vi "gentec-M-Link.Example.vi"() -> ()   [LabVIEW 2014, in "gentec-M-Link - Driver.lvlib"]
uses:
  gentec-M-Link - Driver.lvlib
  Driver/Type Defs/gentec-M-Link.Waveform Averages.ctl
  Driver/Type Defs/gentec-M-Link.Range Queries.ctl
  Driver/Type Defs/gentec-M-Link.Range.ctl
  Driver/Type Defs/gentec-M-Link.Head Attributes.ctl
  Driver/Type Defs/gentec-M-Link.Sensor Type.ctl
  Driver/Type Defs/gentec-M-Link.Trigger Polarity.ctl
  Driver/Type Defs/gentec-M-Link.Trigger Source.ctl
  Driver/Type Defs/gentec-M-Link.Queries with String Answers.ctl
  Driver/Type Defs/gentec-M-Link.Measurement Mode.ctl
panel:
  in  "VISA resource":refnum<visa-resource-name>="visa://pppc069/COM6"
  in  "Action":u32(colorbox)
  in  "Tab Control":T1(tab)
  in  "Get Head connected":bool caption="Check: Head connected?"
  in  "String to send":string
  out "Timeout Test":bool caption="Timeout"
  out "Data read Test":string caption="Data read"
  out "Timeout Head connected":bool caption="Timeout"
  out "Data read Head connected":string caption="Data read"
  out "Head connected?":bool
  in  "Set Block Signal":bool
  in  "Query Head Attributes":bool
  out "Head Attributes":T2={"Firmware"="1.00.00\r\n", "Head Type"="PE3B-Si\r\n", "Head S/N"=501232, "min. Wavelength"=200.0, "max. Wavelength"=1060.0, "Wavelength"=200.0, "Area"=0.0, "Range"=0, "max. Range"=0} {"max. Range" items=["1f", "3f", "10f", "30f", "100f", "300f", "1p", "3p", "10p", "30p", "100p", "300p", "1n", "3n", "10n", "30n", "100n", "300n", "1u", "3u", "10u", "30u", "100u", "300u", "1m", "3m", "10m", "30m", "100m", "300m", "1", "3", "10", "30", "100", "300", "1K", "3K", "10K", "30K", "100K", "300K", "1M", "3M", "10M", "30M", "100M", "300M"]; "Range" items=["1f", "3f", "10f", "30f", "100f", "300f", "1p", "3p", "10p", "30p", "100p", "300p", "1n", "3n", "10n", "30n", "100n", "300n", "1u", "3u", "10u", "30u", "100u", "300u", "1m", "3m", "10m", "30m", "100m", "300m", "1", "3", "10", "30", "100", "300", "1K", "3K", "10K", "30K", "100K", "300K", "1M", "3M", "10M", "30M", "100M", "300M"]}
  out "Any Timeout head Attributes?":bool caption="Timeout"
  out "all Data read":string caption="Data read"
  out "Aswer":string caption="Answer"
  in  "Queries with String Answers":T4="VER"
  in  "Query Cal Lambda":bool
  out "Timeout Cal Lambda":bool caption="Timeout"
  out "Data read Cal Lambda":string caption="Data read"
  in  "Query Sensor Type":bool
  out "Timeout Sensor Type":bool caption="Timeout"
  out "Data read Sensor Type":string caption="Data read"
  out "Sensor Type":T5=2 items=["unknown", "Radiometer", "Joule Meter", "Optical Power", "Thermopyle Power"]
  out "Cal Lambda":i32
  out "Timeout Queries with String Answers":bool caption="Timeout"
  out "Data read  Queries with String Answers":string caption="Data read"
  in  "Get Waveform Averages":bool
  out "Timeout Get Waveform Averages":bool caption="Timeout"
  out "Data read Get Waveform Averages":string caption="Data read"
  in  "Set Waveform Averages":T6 items=["None", "2", "4", "8", "16", "32", "64", "128"]
  out "Timeout Set Waveform Averages":bool caption="Timeout"
  out "Data read Set Waveform Averages":string caption="Data read"
  out "ok Set Waveform Averages":bool caption="ok"
  out "Waveform Averages":T6 items=["None", "2", "4", "8", "16", "32", "64", "128"]
  in  "Set Zero":bool
  out "Range Set Zero":T3 caption="Range" items=["1f", "3f", "10f", "30f", "100f", "300f", "1p", "3p", "10p", "30p", "100p", "300p", "1n", "3n", "10n", "30n", "100n", "300n", "1u", "3u", "10u", "30u", "100u", "300u", "1m", "3m", "10m", "30m", "100m", "300m", "1", "3", "10", "30", "100", "300", "1K", "3K", "10K", "30K", "100K", "300K", "1M", "3M", "10M", "30M", "100M", "300M"]
  out "ok Set Zero":bool caption="ok"
  out "Data Read Set Zero":string caption="Data Read"
  out "Read Timeout Set Zero":bool caption="Timeout"
  out "Max Range Wavelength 2":dbl caption="Offset [V]"
  out "Current Range Wavelength 2":u32 caption="ADC Counts"
  out "Energy evolution":dbl(graph)
  in  "Get current measurement":bool
  out "Energy [J]":dbl format="%_3p"
  in  "Start or stop Data Flow":bool
  out "last measured Energy [J]":dbl format="%_3p"
  out "Success Stop Continuous Mode":bool caption="Success"
  out "Timeout Stop Continuous Mode":bool caption="Timeout"
  out "Data Read Continuous Mode":string caption="Data Read"
  out "Data Read Current Measurement":string
  out "Read Timeout Current Measurement":bool caption="Timeout"
  in  "Set Wavelength":u16 caption="Set Wavelength (nm)"
  out "Min Range Wavelength":T3 caption="Min Range" items=["1f", "3f", "10f", "30f", "100f", "300f", "1p", "3p", "10p", "30p", "100p", "300p", "1n", "3n", "10n", "30n", "100n", "300n", "1u", "3u", "10u", "30u", "100u", "300u", "1m", "3m", "10m", "30m", "100m", "300m", "1", "3", "10", "30", "100", "300", "1K", "3K", "10K", "30K", "100K", "300K", "1M", "3M", "10M", "30M", "100M", "300M"]
  out "Max Range Wavelength":T3 caption="Max Range" items=["1f", "3f", "10f", "30f", "100f", "300f", "1p", "3p", "10p", "30p", "100p", "300p", "1n", "3n", "10n", "30n", "100n", "300n", "1u", "3u", "10u", "30u", "100u", "300u", "1m", "3m", "10m", "30m", "100m", "300m", "1", "3", "10", "30", "100", "300", "1K", "3K", "10K", "30K", "100K", "300K", "1M", "3M", "10M", "30M", "100M", "300M"]
  out "Current Range Wavelength":T3 caption="Current Range" items=["1f", "3f", "10f", "30f", "100f", "300f", "1p", "3p", "10p", "30p", "100p", "300p", "1n", "3n", "10n", "30n", "100n", "300n", "1u", "3u", "10u", "30u", "100u", "300u", "1m", "3m", "10m", "30m", "100m", "300m", "1", "3", "10", "30", "100", "300", "1K", "3K", "10K", "30K", "100K", "300K", "1M", "3M", "10M", "30M", "100M", "300M"]
  out "Corrections Wavelength":bool caption="Corrections"
  out "Read Timeout Set Wavelength":bool caption="Timeout"
  out "Data Read Set Wavelength":string caption="Data Read"
  out "Error Set Wavelength":bool caption="Error"
  out "Min Lambda":i32
  out "Max Lambda":i32
  out "Data Read Set Head Attenuator":string caption="Data Read"
  out "Read Timeout Set Head Attenuator":bool caption="Timeout"
  in  "Set Head Attenuator":bool
  out "Data Read Set Range":string caption="Data Read"
  out "ok Set Autorange?":bool caption="ok?"
  out "Data Read Set Auto Range":string caption="Data Read"
  out "Read Timeout Set Auto Range":bool caption="Timeout"
  in  "Set Auto Range":bool
  in  "Get Range":T7="RNG"
  in  "Set Range":T3 items=["1f", "3f", "10f", "30f", "100f", "300f", "1p", "3p", "10p", "30p", "100p", "300p", "1n", "3n", "10n", "30n", "100n", "300n", "1u", "3u", "10u", "30u", "100u", "300u", "1m", "3m", "10m", "30m", "100m", "300m", "1", "3", "10", "30", "100", "300", "1K", "3K", "10K", "30K", "100K", "300K", "1M", "3M", "10M", "30M", "100M", "300M"]
  out "ok Set Range?":bool caption="ok?"
  out "Read Timeout Set Range":bool caption="Timeout"
  out "Range":T3 items=["1f", "3f", "10f", "30f", "100f", "300f", "1p", "3p", "10p", "30p", "100p", "300p", "1n", "3n", "10n", "30n", "100n", "300n", "1u", "3u", "10u", "30u", "100u", "300u", "1m", "3m", "10m", "30m", "100m", "300m", "1", "3", "10", "30", "100", "300", "1K", "3K", "10K", "30K", "100K", "300K", "1M", "3M", "10M", "30M", "100M", "300M"]
  out "Data Read Get Range":string caption="Data Read"
  out "Read Timeout Get Range":bool caption="Timeout"
  out "Error Get Range":bool caption="Error"
  in  "Set Trigger Level [%]":dbl
  out "ok Set Trigger Level?":bool caption="ok?"
  out "Read Timeout Set Trigger Level":bool caption="Timeout"
  out "Data Read Set Trigger Level":string caption="Data Read"
  in  "Set Trigger Polarity":T8 items=["Falling Edge", "Rising Edge"]
  out "ok Set Trigger Polarity?":bool caption="ok?"
  out "Read Timeout Set Trigger Polarity":bool caption="Timeout"
  out "Data Read Set Trigger Polarity":string caption="Data Read"
  in  "Set Trigger Source":T9 items=["Internal", "External"]
  in  "Get Trigger Level":bool
  out "Trigger Level [%]":dbl
  out "Read Timeout Trigger Level":bool caption="Timeout"
  out "Data Read Trigger Level":string caption="Data Read"
  out "Error Trigger Level":bool caption="Error"
  in  "Set SSE":bool
  out "ok Set SSE?":bool caption="ok?"
  out "Read Timeout Set SSE":bool caption="Timeout"
  out "Data Read Set SSE":string caption="Data Read"
  out "no Thermopyle Head":bool
  in  "Set Anticipation":bool
  out "Data read Set Anticipation":string caption="Data read"
  out "Timeout Set Anticipation":bool caption="Timeout"
  out "ok Anticipation?":bool caption="ok?"
  out "error out":errorcluster
  in  "stop":bool
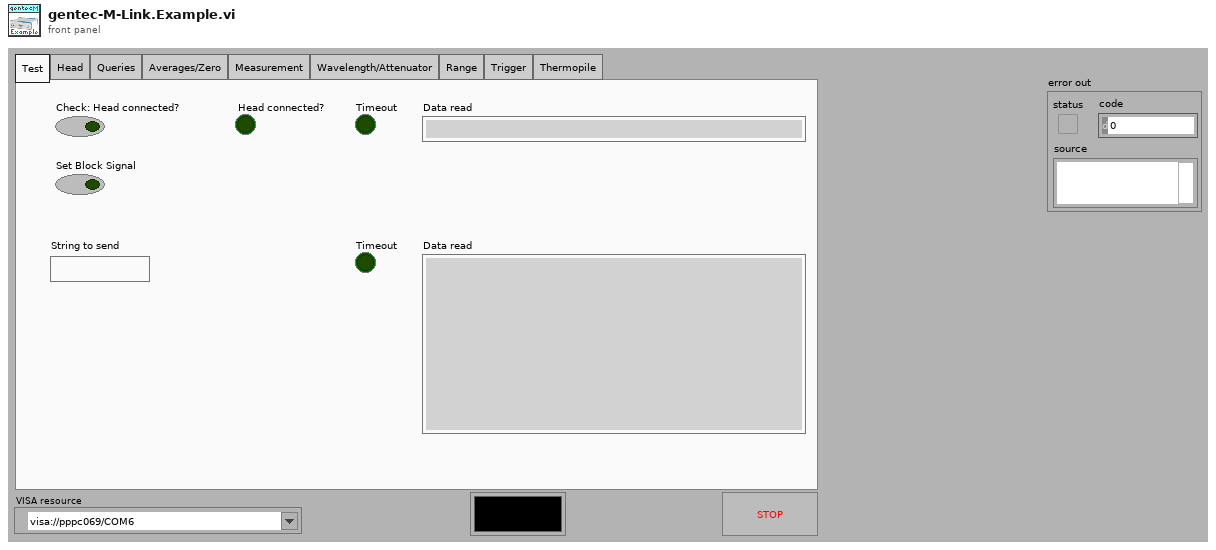
[diagram p1: front panel]
types:
  T1 = enum32{"Test", "Head", "Queries", "Averages/Zero", "Measurement", "Wavelength/Attenuator", "Range", "Trigger", "Thermopile"}
  T2 = typedef "gentec-M-Link - Driver.lvlib/gentec-M-Link.Head Attributes.ctl" = cluster{"Firmware":string, "Head Type":string, "Head S/N":u32, "min. Wavelength":dbl, "max. Wavelength":dbl, "Wavelength":dbl, "Area":dbl, "Range":T3, "max. Range":T3}
  T3 = typedef "gentec-M-Link - Driver.lvlib/gentec-M-Link.Range.ctl" = u16
  T4 = typedef "gentec-M-Link - Driver.lvlib/gentec-M-Link.Queries with String Answers.ctl" = string
  T5 = typedef "gentec-M-Link - Driver.lvlib/gentec-M-Link.Sensor Type.ctl" = u16
  T6 = typedef "gentec-M-Link - Driver.lvlib/gentec-M-Link.Waveform Averages.ctl" = u16
  T7 = typedef "gentec-M-Link - Driver.lvlib/gentec-M-Link.Range Queries.ctl" = string
  T8 = typedef "gentec-M-Link - Driver.lvlib/gentec-M-Link.Trigger Polarity.ctl" = u16
  T9 = typedef "gentec-M-Link - Driver.lvlib/gentec-M-Link.Trigger Source.ctl" = u16
  T10 = typedef "gentec-M-Link - Driver.lvlib/gentec-M-Link.Measurement Mode.ctl" = u16
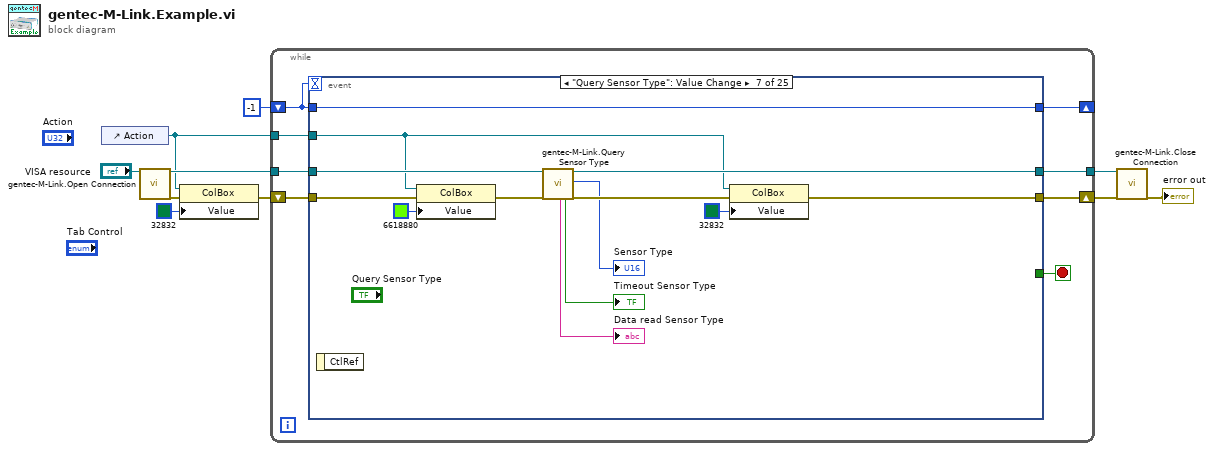
[diagram p0: block diagram]
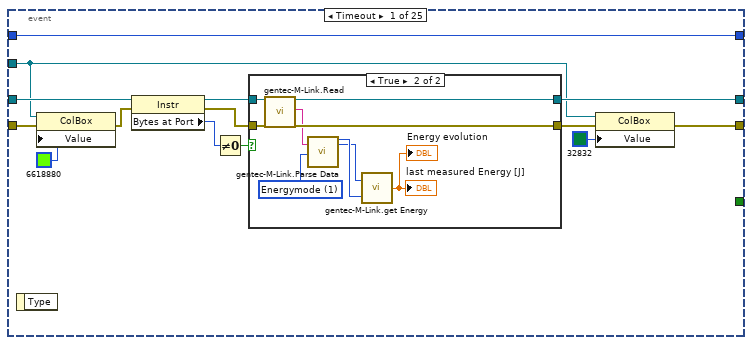
[diagram p2: hidden frame]
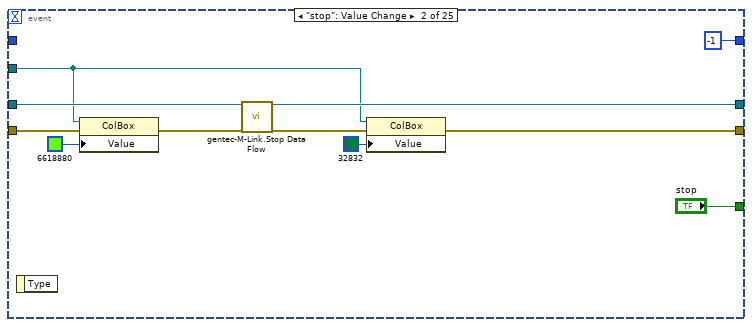
[diagram p4: hidden frame]
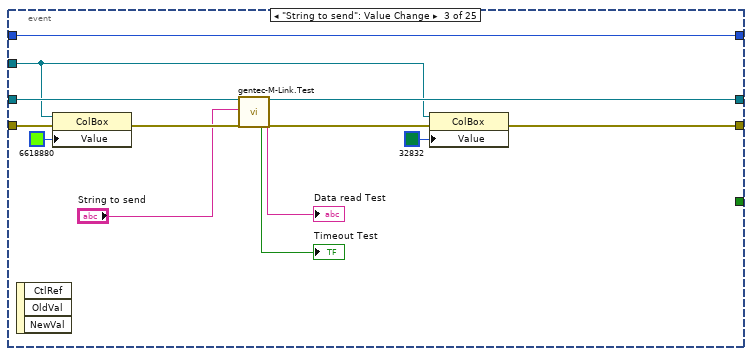
[diagram p5: hidden frame]
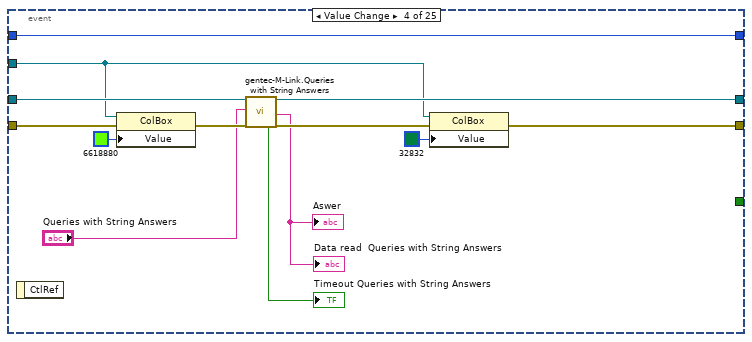
[diagram p6: hidden frame]
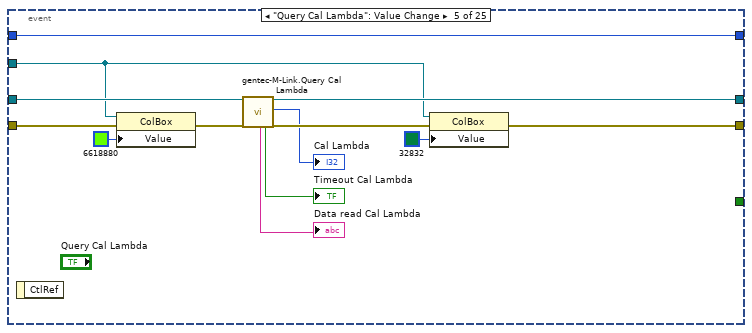
[diagram p7: hidden frame]
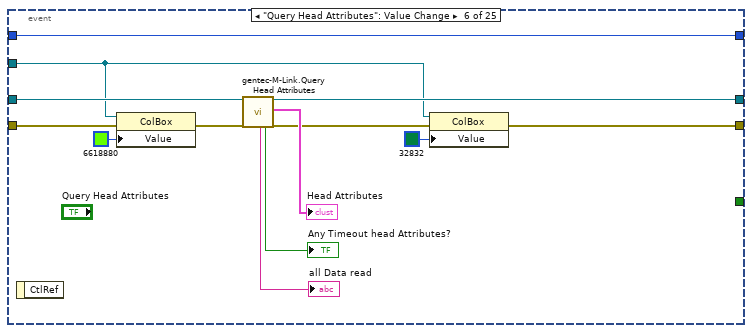
[diagram p8: hidden frame]
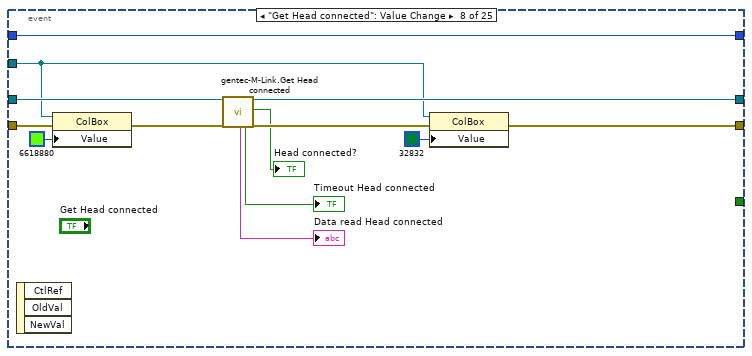
[diagram p9: hidden frame]
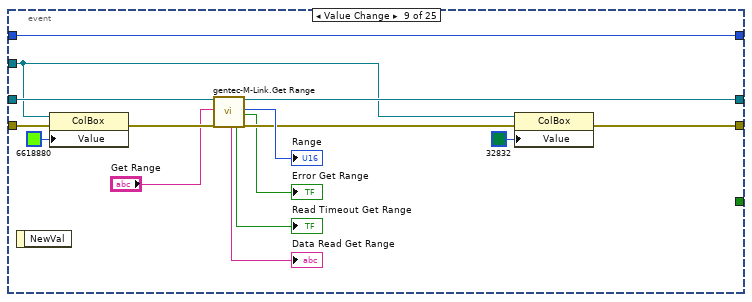
[diagram p10: hidden frame]
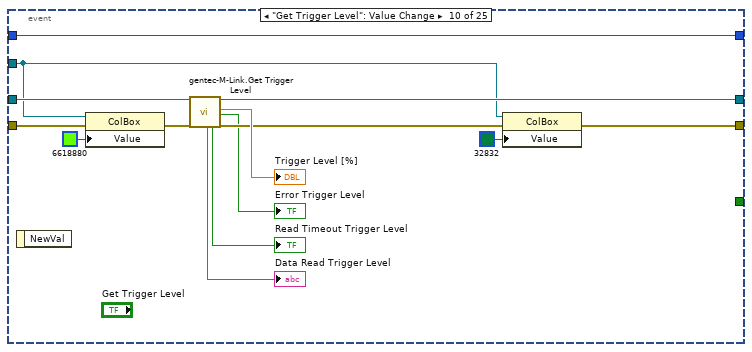
[diagram p11: hidden frame]
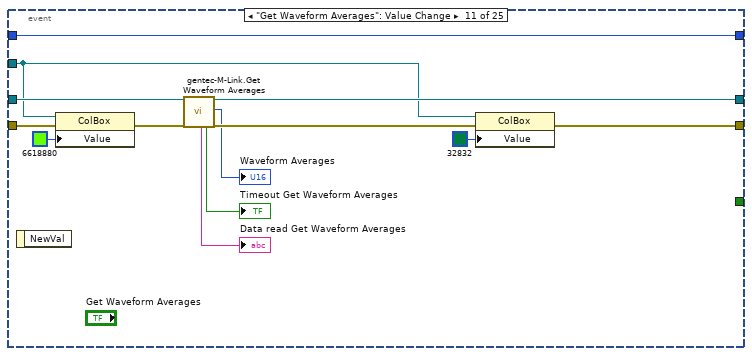
[diagram p12: hidden frame]
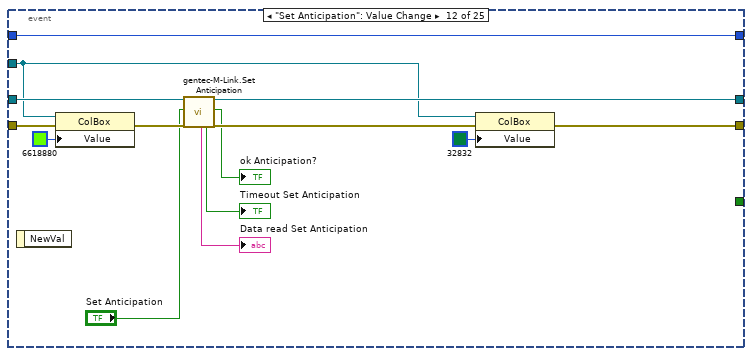
[diagram p13: hidden frame]
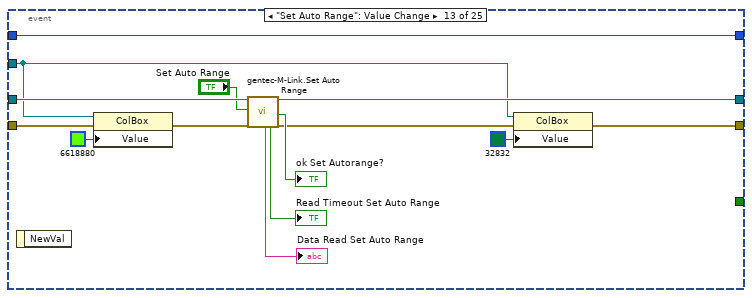
[diagram p14: hidden frame]
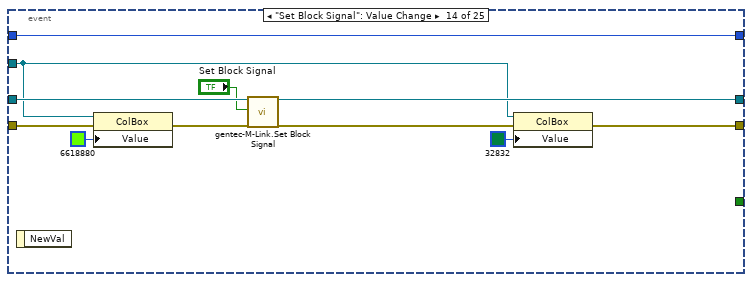
[diagram p15: hidden frame]
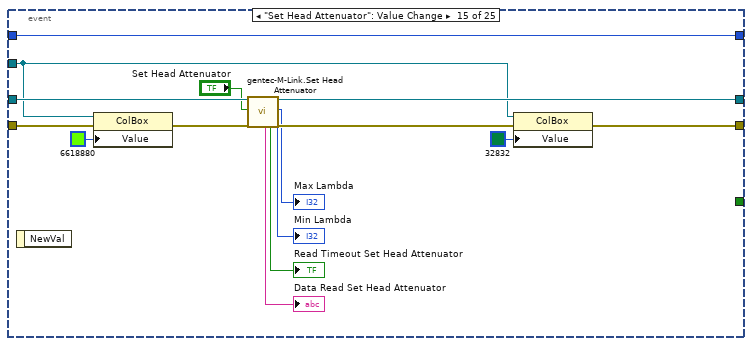
[diagram p16: hidden frame]
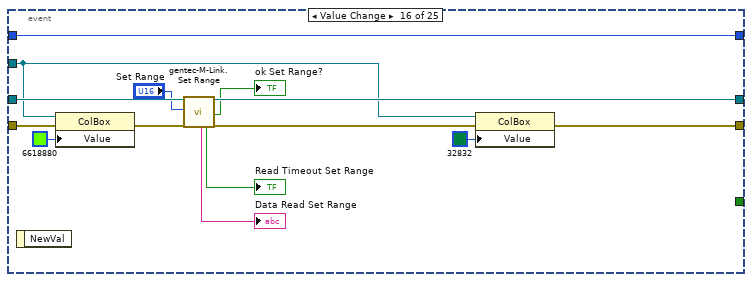
[diagram p17: hidden frame]
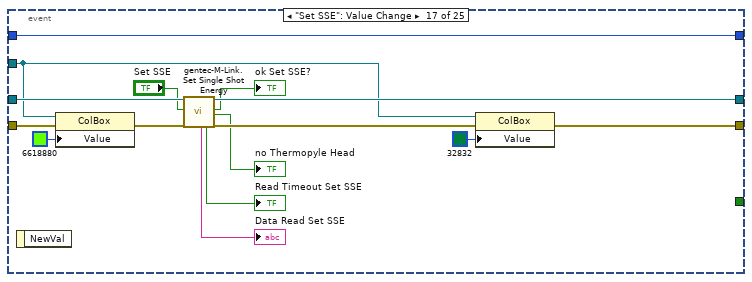
[diagram p18: hidden frame]
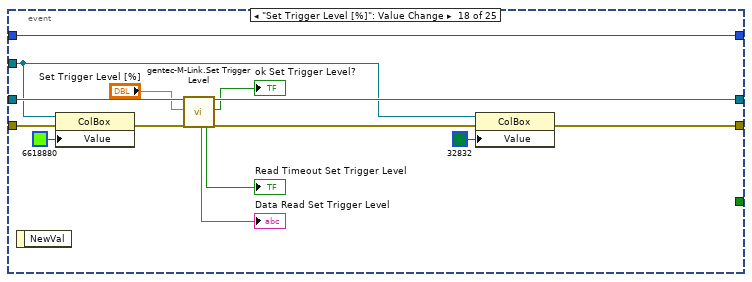
[diagram p19: hidden frame]
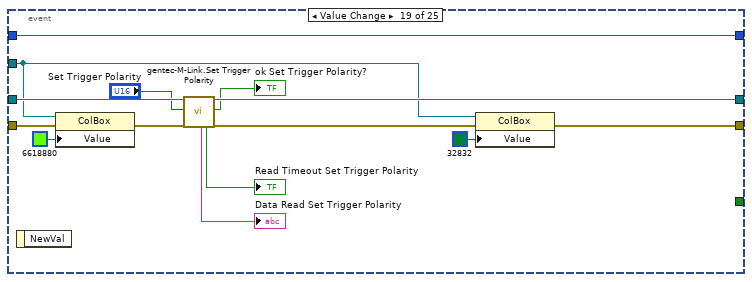
[diagram p20: hidden frame]
diagram:
  n1 = control-ref of="Action"() -> (w3:refnum<vi>)
  n2 = call "gentec-M-Link.Open Connection.vi"("VISA resource (In)"="VISA resource") -> ("VISA resource (Out)"=w5:refnum<visa-resource-name>, "error out"=w4:errorcluster)  [unwired: 17 in]
  n3 = property on="Property Node" class="ColBox"(reference=w3, error in=w4, "Value"=u32 32832 ("Color Box")) -> (error out=w1:errorcluster)  [unwired: 1 out]
  n4 = while {
    tunnel: w5 -> [w17]
    tunnel: [w13] -> w9
    shift-right: [w12] -> w10
    shift-left: w1 -> [w16]
    shift-right: [w14] -> _
    shift-left: -1 -> [w15]
    tunnel: w3 -> [w11]
    stop <- w18 stop-if-true
    n5 = event shown="[6] \"Query Sensor Type\": Value Change" {
      selector: _ -> [_ _ _ _ _ _ _ _ _ _ _ _ _ _ _ _ _ _ _ _ _ _ _ _ _]
      dyn-events: _ -> [_ _ _ _ _ _ _ _ _ _ _ _ _ _ _ _ _ _ _ _ _ _ _ _ _]
      timeout: w15 -> [_ _ _ _ _ _ _ _ _ _ _ _ _ _ _ _ _ _ _ _ _ _ _ _ _]
      tunnel: [_ "stop" _ _ _ _ _ _ _ _ _ _ _ _ _ _ _ _ _ _ _ _ _ _ _] -> w18
      tunnel: w17 -> [w32 w53 w67 w80 w93 w106 w119 w132 w147 w161 w174 w188 w202 w213 w228 w242 w257 w271 w285 w296 w310 w328 w344 w360 w371]
      tunnel: [w28 w52 w66 w79 w92 w105 w118 w131 w146 w160 w173 w187 w201 w212 w227 w241 w256 w270 w284 w295 w309 w326 w343 w359 w370] -> w13
      tunnel: w16 -> [w23 w48 w65 w78 w91 w101 w117 w130 w140 w154 w170 w184 w194 w208 w224 w234 w250 w263 w277 w291 w306 w313 w331 w350 w365]
      tunnel: [w21 w45 w62 w75 w88 w98 w114 w127 w137 w151 w167 w181 w191 w205 w221 w231 w247 w260 w274 w288 w303 w314 w332 w347 w363] -> w12
      tunnel: w15 -> [w26 _ w56 w70 w81 w94 w107 w121 w135 w149 w165 w179 w189 w203 w219 w229 w245 w258 w272 w286 w301 w311 w329 w345 _]
      tunnel: [w26 -1 w56 w70 w81 w94 w107 w121 w135 w149 w165 w179 w189 w203 w219 w229 w245 w258 w272 w286 w301 w311 w329 w345 w368] -> w14
      tunnel: w11 -> [w19 w44 w61 w74 w87 w97 w113 w126 w136 w150 w166 w180 w190 w204 w220 w230 w246 w259 w273 w287 w302 w312 w330 w346 w361]
      event Timeout {
        n6 = event-data() -> ()  [unwired: 1 in, 1 out]
        n7 = property on="Property Node" class="ColBox"(reference=w19, error in=w23, "Value"=u32 6618880 ("Color Box")) -> (error out=w22:errorcluster)  [unwired: 1 out]
        n8 = property class="Instr"(reference=w32, error in=w22) -> (reference out=w29:refnum<visa-resource-name>, error out=w27:errorcluster, "Bytes at Port"=w31:u32)
        n9 = Not Equal To 0?(x=w31) -> (x != 0?=w30:bool)
        n10 = case shown="True" w30 {
          tunnel: w29 -> [w34 w43]
          tunnel: [w34 w42] -> w28
          tunnel: w27 -> [w33 w41]
          tunnel: [w33 w40] -> w20
          frame False {
          }
          frame True {
            w37 = T10 1 items=["other Mode", "Energymode"] ("Measurement")
            n11 = call "gentec-M-Link.Read.vi"("VISA resource (In)"=w43, "error in (no error)"=w41) -> ("VISA resource (Out)"=w42:refnum<visa-resource-name>, "Data Read"=w39:string, "error out"=w40:errorcluster)  [unwired: 13 in, 2 out]
            n12 = call "gentec-M-Link.Parse Data.vi"("Data Bytes"=w39, "Measurement"=w37) -> ("ADC Counts"=w36:u16, "Range"=w35:T3)  [unwired: 13 in, 3 out]
            n13 = call "gentec-M-Link.get Energy.vi"("ADC Counts"=w36, "Range"=w35) -> ("Energy [J]"=→"last measured Energy [J]" →"Energy evolution":dbl)
          }
        }
        n14 = property on="Property Node" class="ColBox"(reference=w19, error in=w20, "Value"=u32 32832 ("Color Box")) -> (error out=w21:errorcluster)  [unwired: 1 out]
      }
      event "stop": Value Change {
        n15 = event-data() -> ()  [unwired: 1 in, 1 out]
        n16 = property on="Property Node" class="ColBox"(reference=w44, error in=w48, "Value"=u32 6618880 ("Color Box")) -> (error out=w47:errorcluster)  [unwired: 1 out]
        n17 = call "gentec-M-Link.Stop Data Flow.vi"("VISA resource In"=w53, "error in (no error)"=w47) -> ("VISA resource Out"=w52:refnum<visa-resource-name>, "error out"=w46:errorcluster)  [unwired: 13 in, 3 out]
        n18 = property on="Property Node" class="ColBox"(reference=w44, error in=w46, "Value"=u32 32832 ("Color Box")) -> (error out=w45:errorcluster)  [unwired: 1 out]
      }
      event "String to send": Value Change {
        n19 = event-data() -> ()  [unwired: 1 in, 3 out]
        n20 = property on="Property Node" class="ColBox"(reference=w61, error in=w65, "Value"=u32 6618880 ("Color Box")) -> (error out=w64:errorcluster)  [unwired: 1 out]
        n21 = call "gentec-M-Link.Test.vi"("VISA resource In"=w67, "Data to Write"="String to send", "error in (no error)"=w64) -> ("Read Timeout"=→"Timeout Test":bool, "VISA resource Out"=w66:refnum<visa-resource-name>, "Data Read"=→"Data read Test":string, "error out"=w63:errorcluster)  [unwired: 13 in]
        n22 = property on="Property Node" class="ColBox"(reference=w61, error in=w63, "Value"=u32 32832 ("Color Box")) -> (error out=w62:errorcluster)  [unwired: 1 out]
      }
      event Value Change {
        n23 = event-data() -> ()  [unwired: 1 in, 1 out]
        n24 = property on="Property Node" class="ColBox"(reference=w74, error in=w78, "Value"=u32 6618880 ("Color Box")) -> (error out=w77:errorcluster)  [unwired: 1 out]
        n25 = call "gentec-M-Link.Queries with String Answers.vi"("VISA resource In"=w80, "Queries with String Answers"="Queries with String Answers", "error in (no error)"=w77) -> ("Read Timeout"=→"Timeout Queries with String Answers":bool, "VISA resource Out"=w79:refnum<visa-resource-name>, "Answer"=→"Data read  Queries with String Answers" →"Aswer":string, "error out"=w76:errorcluster)  [unwired: 13 in]
        n26 = property on="Property Node" class="ColBox"(reference=w74, error in=w76, "Value"=u32 32832 ("Color Box")) -> (error out=w75:errorcluster)  [unwired: 1 out]
      }
      event "Query Cal Lambda": Value Change {
        n27 = event-data() -> ()  [unwired: 1 in, 1 out]
        n28 = property on="Property Node" class="ColBox"(reference=w87, error in=w91, "Value"=u32 6618880 ("Color Box")) -> (error out=w90:errorcluster)  [unwired: 1 out]
        n29 = call "gentec-M-Link.Query Cal Lambda.vi"("VISA resource In"=w93, "error in (no error)"=w90) -> ("Data Read"=→"Data read Cal Lambda":string, "Read Timeout"=→"Timeout Cal Lambda":bool, "VISA resource Out"=w92:refnum<visa-resource-name>, "Cal Lambda"=→"Cal Lambda":i32, "error out"=w89:errorcluster)  [unwired: 13 in]
        n30 = property on="Property Node" class="ColBox"(reference=w87, error in=w89, "Value"=u32 32832 ("Color Box")) -> (error out=w88:errorcluster)  [unwired: 1 out]
      }
      event "Query Head Attributes": Value Change {
        n31 = event-data() -> ()  [unwired: 1 in, 1 out]
        n32 = property on="Property Node" class="ColBox"(reference=w97, error in=w101, "Value"=u32 6618880 ("Color Box")) -> (error out=w100:errorcluster)  [unwired: 1 out]
        n33 = call "gentec-M-Link.Query Head Attributes.vi"("VISA resource In"=w106, "error in (no error)"=w100) -> ("all Data read"=→"all Data read":string, "Any Timeout?"=→"Any Timeout head Attributes?":bool, "VISA resource Out"=w105:refnum<visa-resource-name>, "Head Attributes"=→"Head Attributes":T2, "error out"=w99:errorcluster)  [unwired: 13 in]
        n34 = property on="Property Node" class="ColBox"(reference=w97, error in=w99, "Value"=u32 32832 ("Color Box")) -> (error out=w98:errorcluster)  [unwired: 1 out]
      }
      event "Query Sensor Type": Value Change {
        n35 = event-data() -> ()  [unwired: 1 in, 1 out]
        n36 = property on="Property Node" class="ColBox"(reference=w113, error in=w117, "Value"=u32 6618880 ("Color Box")) -> (error out=w116:errorcluster)  [unwired: 1 out]
        n37 = call "gentec-M-Link.Query Sensor Type.vi"("VISA resource In"=w119, "error in (no error)"=w116) -> ("Data Read"=→"Data read Sensor Type":string, "Read Timeout"=→"Timeout Sensor Type":bool, "VISA resource Out"=w118:refnum<visa-resource-name>, "Sensor Type"=→"Sensor Type":T5, "error out"=w115:errorcluster)  [unwired: 13 in]
        n38 = property on="Property Node" class="ColBox"(reference=w113, error in=w115, "Value"=u32 32832 ("Color Box")) -> (error out=w114:errorcluster)  [unwired: 1 out]
      }
      event "Get Head connected": Value Change {
        n39 = event-data() -> ()  [unwired: 1 in, 3 out]
        n40 = property on="Property Node" class="ColBox"(reference=w126, error in=w130, "Value"=u32 6618880 ("Color Box")) -> (error out=w129:errorcluster)  [unwired: 1 out]
        n41 = call "gentec-M-Link.Get Head connected.vi"("VISA resource In"=w132, "error in (no error)"=w129) -> ("Data Read"=→"Data read Head connected":string, "Read Timeout"=→"Timeout Head connected":bool, "VISA resource Out"=w131:refnum<visa-resource-name>, "Head connected?"=→"Head connected?":bool, "error out"=w128:errorcluster)  [unwired: 13 in]
        n42 = property on="Property Node" class="ColBox"(reference=w126, error in=w128, "Value"=u32 32832 ("Color Box")) -> (error out=w127:errorcluster)  [unwired: 1 out]
      }
      event Value Change {
        n43 = event-data() -> ()  [unwired: 1 in, 1 out]
        n44 = property on="Property Node" class="ColBox"(reference=w136, error in=w140, "Value"=u32 6618880 ("Color Box")) -> (error out=w139:errorcluster)  [unwired: 1 out]
        n45 = call "gentec-M-Link.Get Range.vi"("VISA resource In"=w147, "Range Queries"="Get Range", "error in (no error)"=w139) -> ("Data Read"=→"Data Read Get Range":string, "Read Timeout"=→"Read Timeout Get Range":bool, "VISA resource Out"=w146:refnum<visa-resource-name>, "Range"=→"Range":T3, "Error"=→"Error Get Range":bool, "error out"=w138:errorcluster)  [unwired: 11 in]
        n46 = property on="Property Node" class="ColBox"(reference=w136, error in=w138, "Value"=u32 32832 ("Color Box")) -> (error out=w137:errorcluster)  [unwired: 1 out]
      }
      event "Get Trigger Level": Value Change {
        n47 = event-data() -> ()  [unwired: 1 in, 1 out]
        n48 = property on="Property Node" class="ColBox"(reference=w150, error in=w154, "Value"=u32 6618880 ("Color Box")) -> (error out=w153:errorcluster)  [unwired: 1 out]
        n49 = call "gentec-M-Link.Get Trigger Level.vi"("VISA resource In"=w161, "error in (no error)"=w153) -> ("Data Read"=→"Data Read Trigger Level":string, "Read Timeout"=→"Read Timeout Trigger Level":bool, "VISA resource Out"=w160:refnum<visa-resource-name>, "Trigger Level [%]"=→"Trigger Level [%]":dbl, "Error"=→"Error Trigger Level":bool, "error out"=w152:errorcluster)  [unwired: 12 in]
        n50 = property on="Property Node" class="ColBox"(reference=w150, error in=w152, "Value"=u32 32832 ("Color Box")) -> (error out=w151:errorcluster)  [unwired: 1 out]
      }
      event "Get Waveform Averages": Value Change {
        n51 = event-data() -> ()  [unwired: 1 in, 1 out]
        n52 = property on="Property Node" class="ColBox"(reference=w166, error in=w170, "Value"=u32 6618880 ("Color Box")) -> (error out=w169:errorcluster)  [unwired: 1 out]
        n53 = call "gentec-M-Link.Get Waveform Averages.vi"("VISA resource In"=w174, "error in (no error)"=w169) -> ("Data Read"=→"Data read Get Waveform Averages":string, "Read Timeout"=→"Timeout Get Waveform Averages":bool, "VISA resource Out"=w173:refnum<visa-resource-name>, "Waveform Averages"=→"Waveform Averages":T6, "error out"=w168:errorcluster)  [unwired: 13 in]
        n54 = property on="Property Node" class="ColBox"(reference=w166, error in=w168, "Value"=u32 32832 ("Color Box")) -> (error out=w167:errorcluster)  [unwired: 1 out]
      }
      event "Set Anticipation": Value Change {
        n55 = event-data() -> ()  [unwired: 1 in, 1 out]
        n56 = property on="Property Node" class="ColBox"(reference=w180, error in=w184, "Value"=u32 6618880 ("Color Box")) -> (error out=w183:errorcluster)  [unwired: 1 out]
        n57 = call "gentec-M-Link.Set Anticipation.vi"("VISA resource In"=w188, "Enable Anticipation"="Set Anticipation", "error in (no error)"=w183) -> ("Data Read"=→"Data read Set Anticipation":string, "Read Timeout"=→"Timeout Set Anticipation":bool, "VISA resource Out"=w187:refnum<visa-resource-name>, "Success"=→"ok Anticipation?":bool, "error out"=w182:errorcluster)  [unwired: 12 in]
        n58 = property on="Property Node" class="ColBox"(reference=w180, error in=w182, "Value"=u32 32832 ("Color Box")) -> (error out=w181:errorcluster)  [unwired: 1 out]
      }
      event "Set Auto Range": Value Change {
        n59 = event-data() -> ()  [unwired: 1 in, 1 out]
        n60 = property on="Property Node" class="ColBox"(reference=w190, error in=w194, "Value"=u32 6618880 ("Color Box")) -> (error out=w193:errorcluster)  [unwired: 1 out]
        n61 = call "gentec-M-Link.Set Auto Range.vi"("VISA resource In"=w202, "Auto Range"="Set Auto Range", "error in (no error)"=w193) -> ("Data Read"=→"Data Read Set Auto Range":string, "Read Timeout"=→"Read Timeout Set Auto Range":bool, "VISA resource Out"=w201:refnum<visa-resource-name>, "Success"=→"ok Set Autorange?":bool, "error out"=w192:errorcluster)  [unwired: 12 in]
        n62 = property on="Property Node" class="ColBox"(reference=w190, error in=w192, "Value"=u32 32832 ("Color Box")) -> (error out=w191:errorcluster)  [unwired: 1 out]
      }
      event "Set Block Signal": Value Change {
        n63 = event-data() -> ()  [unwired: 1 in, 1 out]
        n64 = property on="Property Node" class="ColBox"(reference=w204, error in=w208, "Value"=u32 6618880 ("Color Box")) -> (error out=w207:errorcluster)  [unwired: 1 out]
        n65 = call "gentec-M-Link.Set Block Signal.vi"("VISA resource In"=w213, "Block Signal"="Set Block Signal", "error in (no error)"=w207) -> ("VISA resource Out"=w212:refnum<visa-resource-name>, "error out"=w206:errorcluster)  [unwired: 15 in]
        n66 = property on="Property Node" class="ColBox"(reference=w204, error in=w206, "Value"=u32 32832 ("Color Box")) -> (error out=w205:errorcluster)  [unwired: 1 out]
      }
      event "Set Head Attenuator": Value Change {
        n67 = event-data() -> ()  [unwired: 1 in, 1 out]
        n68 = property on="Property Node" class="ColBox"(reference=w220, error in=w224, "Value"=u32 6618880 ("Color Box")) -> (error out=w223:errorcluster)  [unwired: 1 out]
        n69 = call "gentec-M-Link.Set Head Attenuator.vi"("VISA resource In"=w228, "Set Head Attenuator"="Set Head Attenuator", "error in (no error)"=w223) -> ("Data Read"=→"Data Read Set Head Attenuator":string, "Read Timeout"=→"Read Timeout Set Head Attenuator":bool, "VISA resource Out"=w227:refnum<visa-resource-name>, "Max Lambda"=→"Max Lambda":i32, "Min Lambda"=→"Min Lambda":i32, "error out"=w222:errorcluster)  [unwired: 11 in]
        n70 = property on="Property Node" class="ColBox"(reference=w220, error in=w222, "Value"=u32 32832 ("Color Box")) -> (error out=w221:errorcluster)  [unwired: 1 out]
      }
      event Value Change {
        n71 = event-data() -> ()  [unwired: 1 in, 1 out]
        n72 = property on="Property Node" class="ColBox"(reference=w230, error in=w234, "Value"=u32 6618880 ("Color Box")) -> (error out=w233:errorcluster)  [unwired: 1 out]
        n73 = call "gentec-M-Link.Set Range.vi"("VISA resource In"=w242, "Range"="Set Range", "error in (no error)"=w233) -> ("Data Read"=→"Data Read Set Range":string, "Read Timeout"=→"Read Timeout Set Range":bool, "VISA resource Out"=w241:refnum<visa-resource-name>, "Success"=→"ok Set Range?":bool, "error out"=w232:errorcluster)  [unwired: 12 in]
        n74 = property on="Property Node" class="ColBox"(reference=w230, error in=w232, "Value"=u32 32832 ("Color Box")) -> (error out=w231:errorcluster)  [unwired: 1 out]
      }
      event "Set SSE": Value Change {
        n75 = event-data() -> ()  [unwired: 1 in, 1 out]
        n76 = property on="Property Node" class="ColBox"(reference=w246, error in=w250, "Value"=u32 6618880 ("Color Box")) -> (error out=w249:errorcluster)  [unwired: 1 out]
        n77 = call "gentec-M-Link.Set Single Shot Energy.vi"("VISA resource In"=w257, "Enable Single Shot Energy"="Set SSE", "error in (no error)"=w249) -> ("Data Read"=→"Data Read Set SSE":string, "Read Timeout"=→"Read Timeout Set SSE":bool, "VISA resource Out"=w256:refnum<visa-resource-name>, "Success"=→"ok Set SSE?":bool, "no Thermopyle Head"=→"no Thermopyle Head":bool, "error out"=w248:errorcluster)  [unwired: 11 in]
        n78 = property on="Property Node" class="ColBox"(reference=w246, error in=w248, "Value"=u32 32832 ("Color Box")) -> (error out=w247:errorcluster)  [unwired: 1 out]
      }
      event "Set Trigger Level [%]": Value Change {
        n79 = event-data() -> ()  [unwired: 1 in, 1 out]
        n80 = property on="Property Node" class="ColBox"(reference=w259, error in=w263, "Value"=u32 6618880 ("Color Box")) -> (error out=w262:errorcluster)  [unwired: 1 out]
        n81 = call "gentec-M-Link.Set Trigger Level.vi"("VISA resource In"=w271, "Trigger Level [%]"="Set Trigger Level [%]", "error in (no error)"=w262) -> ("Data Read"=→"Data Read Set Trigger Level":string, "Read Timeout"=→"Read Timeout Set Trigger Level":bool, "VISA resource Out"=w270:refnum<visa-resource-name>, "Success"=→"ok Set Trigger Level?":bool, "error out"=w261:errorcluster)  [unwired: 12 in]
        n82 = property on="Property Node" class="ColBox"(reference=w259, error in=w261, "Value"=u32 32832 ("Color Box")) -> (error out=w260:errorcluster)  [unwired: 1 out]
      }
      event Value Change {
        n83 = event-data() -> ()  [unwired: 1 in, 1 out]
        n84 = property on="Property Node" class="ColBox"(reference=w273, error in=w277, "Value"=u32 6618880 ("Color Box")) -> (error out=w276:errorcluster)  [unwired: 1 out]
        n85 = call "gentec-M-Link.Set Trigger Polarity.vi"("VISA resource In"=w285, "Trigger Polarity"="Set Trigger Polarity", "error in (no error)"=w276) -> ("Data Read"=→"Data Read Set Trigger Polarity":string, "Read Timeout"=→"Read Timeout Set Trigger Polarity":bool, "VISA resource Out"=w284:refnum<visa-resource-name>, "Success"=→"ok Set Trigger Polarity?":bool, "error out"=w275:errorcluster)  [unwired: 12 in]
        n86 = property on="Property Node" class="ColBox"(reference=w273, error in=w275, "Value"=u32 32832 ("Color Box")) -> (error out=w274:errorcluster)  [unwired: 1 out]
      }
      event Value Change {
        n87 = event-data() -> ()  [unwired: 1 in, 1 out]
        n88 = property on="Property Node" class="ColBox"(reference=w287, error in=w291, "Value"=u32 6618880 ("Color Box")) -> (error out=w290:errorcluster)  [unwired: 1 out]
        n89 = call "gentec-M-Link.Set Trigger Source.vi"("VISA resource In"=w296, "Trigger Source"="Set Trigger Source", "error in (no error)"=w290) -> ("VISA resource Out"=w295:refnum<visa-resource-name>, "error out"=w289:errorcluster)  [unwired: 15 in]
        n90 = property on="Property Node" class="ColBox"(reference=w287, error in=w289, "Value"=u32 32832 ("Color Box")) -> (error out=w288:errorcluster)  [unwired: 1 out]
      }
      event Value Change {
        n91 = event-data() -> ()  [unwired: 1 in, 1 out]
        n92 = property on="Property Node" class="ColBox"(reference=w302, error in=w306, "Value"=u32 6618880 ("Color Box")) -> (error out=w305:errorcluster)  [unwired: 1 out]
        n93 = call "gentec-M-Link.Set Waveform Averages.vi"("VISA resource In"=w310, "Waveform Averages"="Set Waveform Averages", "error in (no error)"=w305) -> ("Data Read"=→"Data read Set Waveform Averages":string, "Read Timeout"=→"Timeout Set Waveform Averages":bool, "VISA resource Out"=w309:refnum<visa-resource-name>, "Success"=→"ok Set Waveform Averages":bool, "error out"=w304:errorcluster)  [unwired: 12 in]
        n94 = property on="Property Node" class="ColBox"(reference=w302, error in=w304, "Value"=u32 32832 ("Color Box")) -> (error out=w303:errorcluster)  [unwired: 1 out]
      }
      event "Set Wavelength": Value Change {
        n95 = event-data() -> ()  [unwired: 1 in, 1 out]
        n96 = property on="Property Node" class="ColBox"(reference=w312, error in=w313, "Value"=u32 6618880 ("Color Box")) -> (error out=w316:errorcluster)  [unwired: 1 out]
        n97 = call "gentec-M-Link.Set Wavelength.vi"("VISA resource In"=w328, "Lambda"="Set Wavelength", "error in (no error)"=w316) -> ("Data Read"=→"Data Read Set Wavelength":string, "Error"=→"Error Set Wavelength":bool, "Read Timeout"=→"Read Timeout Set Wavelength":bool, "VISA resource Out"=w326:refnum<visa-resource-name>, "Min Range"=→"Min Range Wavelength":T3, "Max Range"=→"Max Range Wavelength":T3, "Current Range"=→"Current Range Wavelength":T3, "Corrections"=→"Corrections Wavelength":bool, "error out"=w315:errorcluster)  [unwired: 8 in]
        n98 = property on="Property Node" class="ColBox"(reference=w312, error in=w315, "Value"=u32 32832 ("Color Box")) -> (error out=w314:errorcluster)  [unwired: 1 out]
      }
      event "Set Zero": Value Change {
        n99 = event-data() -> ()  [unwired: 1 in, 1 out]
        n100 = property on="Property Node" class="ColBox"(reference=w330, error in=w331, "Value"=u32 6618880 ("Color Box")) -> (error out=w334:errorcluster)  [unwired: 1 out]
        n101 = call "gentec-M-Link.Set Zero.vi"("VISA resource (In)"=w344, "error in (no error)"=w334) -> ("Data Read"=→"Data Read Set Zero":string, "Read Timeout"=→"Read Timeout Set Zero":bool, "VISA resource (Out)"=w343:refnum<visa-resource-name>, "Range"=→"Range Set Zero":T3, "Offset [V]"=→"Max Range Wavelength 2":dbl, "ADC counts"=→"Current Range Wavelength 2":u32, "Success"=→"ok Set Zero":bool, "error out"=w333:errorcluster)  [unwired: 10 in]
        n102 = property on="Property Node" class="ColBox"(reference=w330, error in=w333, "Value"=u32 32832 ("Color Box")) -> (error out=w332:errorcluster)  [unwired: 1 out]
      }
      event "Get current measurement": Value Change {
        w358 = T10 1 items=["other Mode", "Energymode"] ("Mode")
        n103 = event-data() -> ()  [unwired: 1 in, 1 out]
        n104 = property on="Property Node" class="ColBox"(reference=w346, error in=w350, "Value"=u32 6618880 ("Color Box")) -> (error out=w349:errorcluster)  [unwired: 1 out]
        n105 = call "gentec-M-Link.Current Measurement.vi"("VISA resource In"=w360, "Measurement"=w358, "error in (no error)"=w349) -> ("Data Read"=→"Data Read Current Measurement":string, "Read Timeout"=→"Read Timeout Current Measurement":bool, "VISA resource Out"=w359:refnum<visa-resource-name>, "Range"=w355:T3, "ADC Counts"=w356:u16, "error out"=w348:errorcluster)  [unwired: 7 in, 4 out]
        n106 = call "gentec-M-Link.get Energy.vi"("ADC Counts"=w356, "Range"=w355) -> ("Energy [J]"=→"Energy [J]":dbl)
        n107 = property on="Property Node" class="ColBox"(reference=w346, error in=w348, "Value"=u32 32832 ("Color Box")) -> (error out=w347:errorcluster)  [unwired: 1 out]
      }
      event "Start or stop Data Flow": Value Change {
        n108 = event-data() -> ()  [unwired: 1 in, 1 out]
        n109 = property on="Property Node" class="ColBox"(reference=w361, error in=w365, "Value"=u32 6618880 ("Color Box")) -> (error out=w364:errorcluster)  [unwired: 1 out]
        n110 = case shown="True" "Start or stop Data Flow" {
          tunnel: w371 -> [w379 w384]
          tunnel: [w377 w383] -> w370
          tunnel: [w376 w382] -> w362
          tunnel: w364 -> [w378 w381]
          tunnel: [-1 50] -> w368
          frame False {
            n111 = call "gentec-M-Link.Stop Data Flow.vi"("VISA resource In"=w379, "error in (no error)"=w378) -> ("Data Read"=→"Data Read Continuous Mode":string, "Read Timeout"=→"Timeout Stop Continuous Mode":bool, "VISA resource Out"=w377:refnum<visa-resource-name>, "Success"=→"Success Stop Continuous Mode":bool, "error out"=w376:errorcluster)  [unwired: 13 in]
          }
          frame True {
            n112 = call "gentec-M-Link.Start Data Flow.vi"("VISA resource In"=w384, "error in (no error)"=w381) -> ("VISA resource Out"=w383:refnum<visa-resource-name>, "error out"=w382:errorcluster)  [unwired: 16 in]
          }
        }
        n113 = property on="Property Node" class="ColBox"(reference=w361, error in=w362, "Value"=u32 32832 ("Color Box")) -> (error out=w363:errorcluster)  [unwired: 1 out]
      }
    }
  }
  n114 = call "gentec-M-Link.Close Connection.vi"("VISA resource In"=w9, "error in (no error)"=w10) -> ("error out"=→"error out":errorcluster)  [unwired: 17 in]
